vi "XSP3_ControlEraseData.vi"(6 "Erase":enum16{"OFF", "ON"}(ring) caption="ControlErase", 8 "ErrorIn":errorcluster, 11 "ProcessIn":string="XSPRESS3-EXAMPLE" caption="ProcessName") -> (0 "ErrorOut":errorcluster, 2 "Status":bool, 3 "ProcessOut":string caption="ProcessName")   [LabVIEW 2010]
uses:
  Program Files/National Instruments/LabVIEW 2017/user.lib/caLab/Private/Put_I16_PV.vi
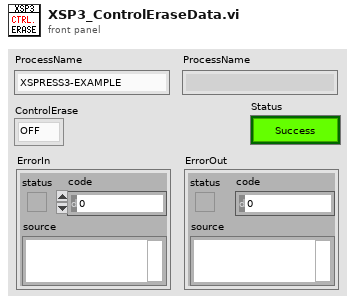
[diagram p1: front panel]
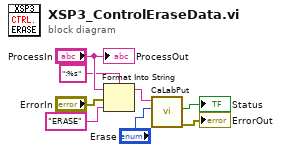
[diagram p0: block diagram]
diagram:
  n1 = Format Into String(format string=":%s" ("PV"), initial string="ProcessIn", error in="ErrorIn", "ERASE" ("PV")) -> (resulting string=w4:string)  [unwired: 1 out]
  n2 = call-poly "CaLabPut.vi"("Value"="Erase", "PV Name"=w4) -> ("Error out"=→"ErrorOut":errorcluster, "Status"=→"Status":bool)  [unwired: 6 in, 2 out]
  "ProcessOut" <- "ProcessIn"
